vi "UI Closed.vi"(0 "Model Base in":refnum<class "Model Base.lvclass">, 11 "error in (no error)":errorcluster) -> (4 "Model Base out":refnum<class "Model Base.lvclass">, 15 "error out":errorcluster)   [LabVIEW 2023, in "Model Base.lvlib" / "Model Base.lvclass"]
uses:
  Model Base.lvclass
  Model Base.lvclass/Model Base.ctl
  <vilib>/ActorFramework/Stop Msg/Stop Msg.lvclass
  <vilib>/ActorFramework/Actor/Actor.lvclass
  C:/Program Files/National Instruments/LabVIEW 2023/vi.lib/ActorFramework/Actor/Actor.lvclass
  C:/Users/bhaghyaraj/Trainings/NI Actor Frameowork/SDLC/Model Base/Model Base/Model Base.lvclass
  C:/Users/bhaghyaraj/Trainings/NI Actor Frameowork/SDLC/Interfaces/Model Base/Incoming Model Base Interface.lvclass
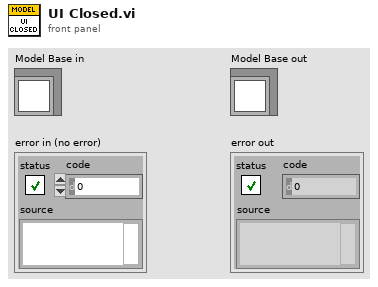
[diagram p1: front panel]
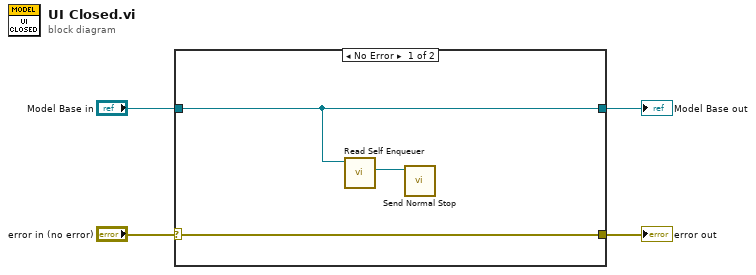
[diagram p0: block diagram]
diagram:
  n1 = case shown="No Error" "error in (no error)" {
    selector: "error in (no error)" -> [w7 w9]
    tunnel: [w7 w9] -> w3
    tunnel: [w5 w8] -> w2
    tunnel: "Model Base in" -> [w5 w8]
    frame No Error {
      n2 = call <vilib>:"Read Self Enqueuer.vi"("Actor"=w5) -> ("Self Enqueuer"=w6:refnum<class "Message Enqueuer.lvclass">)  [unwired: 10 in]
      n3 = call <vilib>:"Send Normal Stop.vi"("Message Enqueuer"=w6) -> ()  [unwired: 10 in, 1 out]
    }
    frame Error {
    }
  }
  "error out" <- w3
  "Model Base out" <- w2
